vi "writegraph_NEW.vi"(3 "FromPLC":string[][](array[string]), 4 "Numeric":i16, 5 "FromMotes":string[][](array[string])) -> ()   [LabVIEW 2011]
uses:
  Dependencies/global.vi
panel:
  out "Actuation Values":T1(graph)
  out "AC":dbl
  out "Radiator":dbl
  out "FreshAirInlet":dbl
  out "OutdoorTemp":dbl
  out "IndoorTemp":dbl
  out "Humidity":dbl(graph)
  out "Temperature":cluster{"IndoorTemp":dbl, " OutdoorTemp":dbl}(graph)
  out "CO2":dbl(graph)
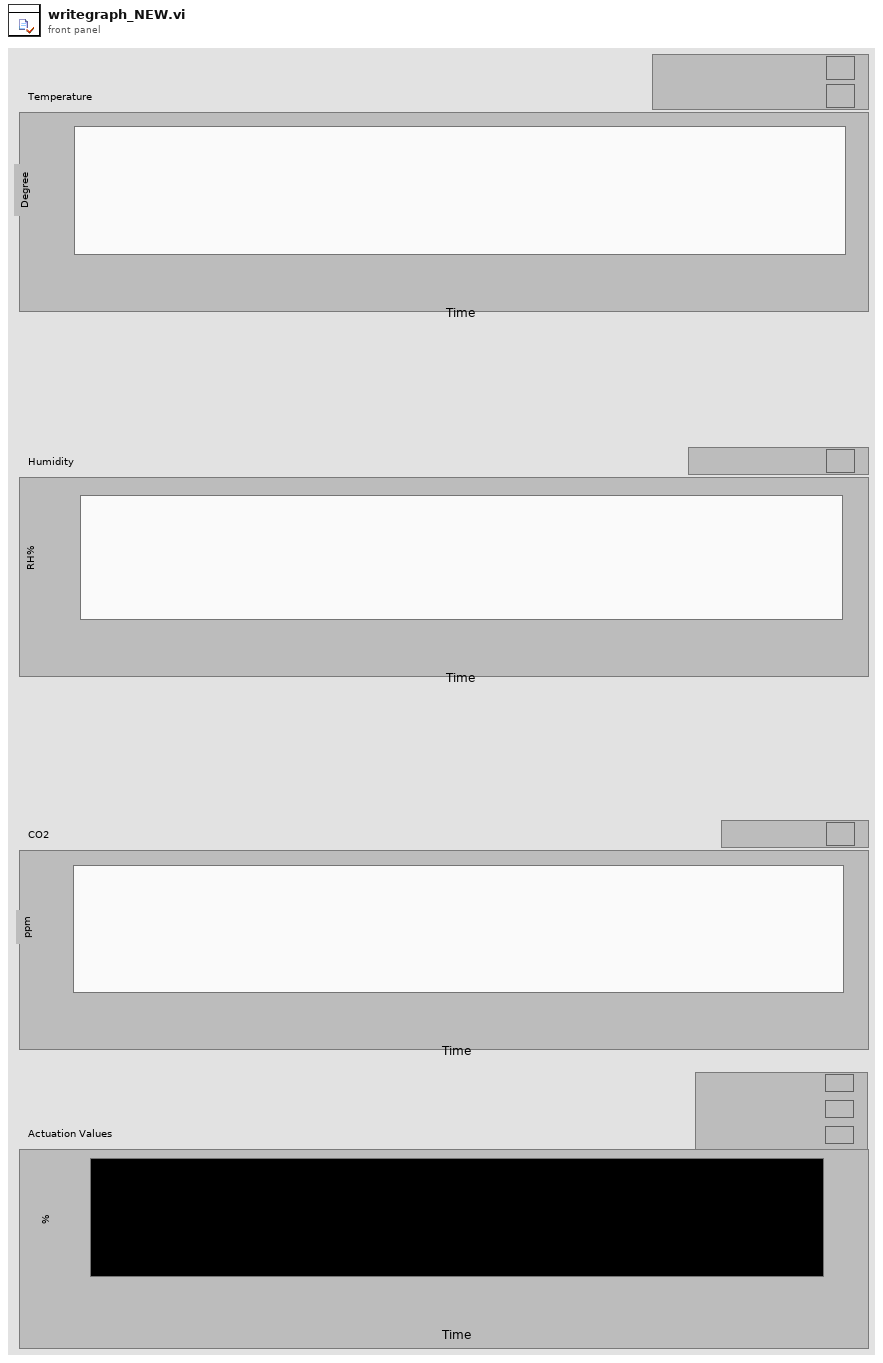
[diagram p1: front panel]
types:
  T1 = cluster{"FreshAirInlet":dbl, "Radiator":dbl, "AC":dbl}
  T2 = typedef "imagedata.ctl" = cluster{"image type":i32, "image depth":i32, "image":u8[], "mask":u8[], "colors":u32[], "Rectangle":cluster{"left":i16, "top":i16, "right":i16, "bottom":i16}}
  T3 = cluster{"FreshAirInlet":dbl, "Radiator":dbl, "AC":dbl}[]
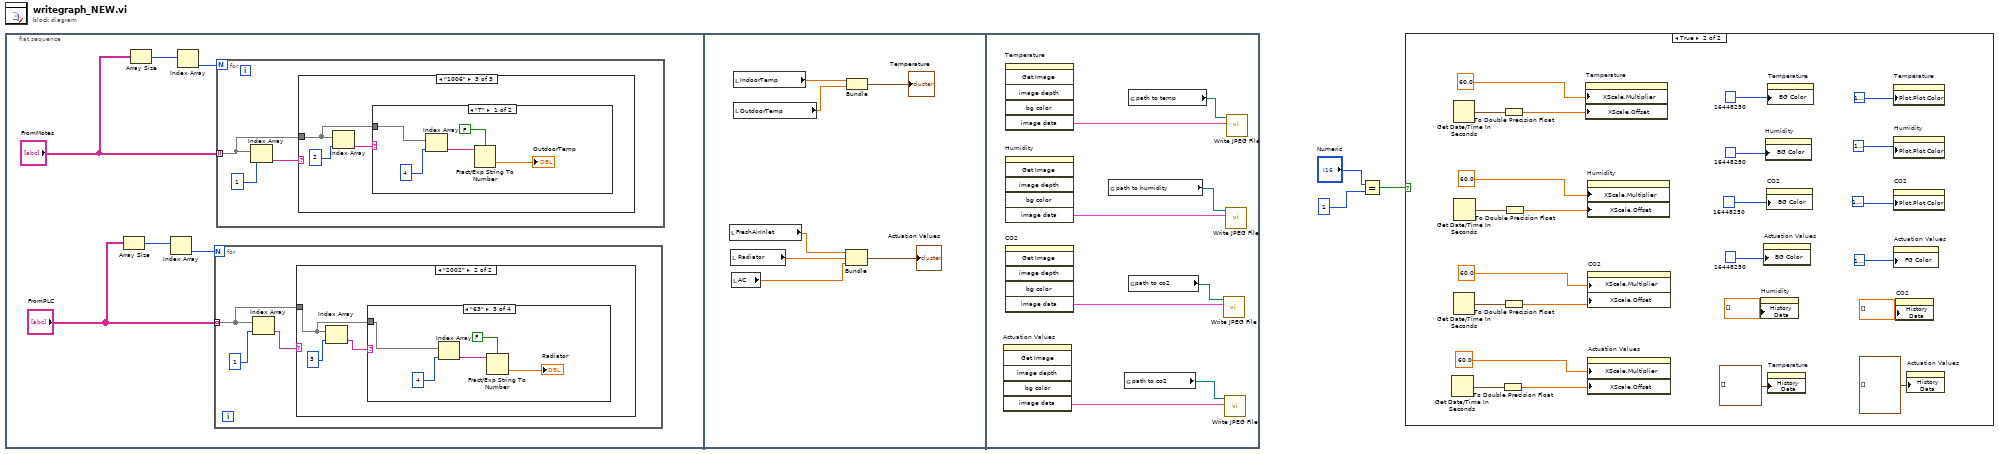
[diagram p0: block diagram]
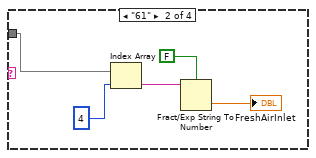
[diagram p4: hidden frame]
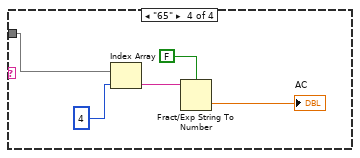
[diagram p5: hidden frame]
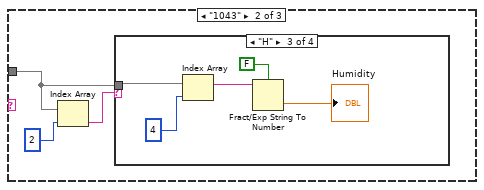
[diagram p7: hidden frame]
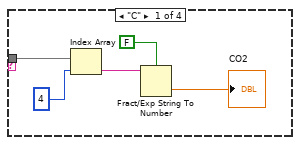
[diagram p8: hidden frame]
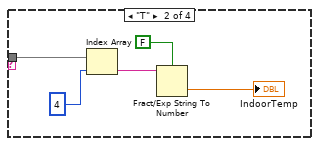
[diagram p9: hidden frame]
diagram:
  n1 = flat-sequence {
    frame #0 {
      n2 = Array Size(array="FromPLC") -> (size(s)=w6:i32[])
      n3 = Array Size(array="FromMotes") -> (size(s)=w9:i32[])
      n4 = Index Array(array=w6) -> (element=w5:i32)  [unwired: 1 in]
      n5 = Index Array(array=w9) -> (element=w8:i32)  [unwired: 1 in]
      n6 = for {
        N: w5 -> [_]
        tunnel: "FromPLC" -> [w10] mode=indexing
        n7 = Index Array(array=w10, index=1) -> (element=w11:string)
        n8 = case shown="\"2002\"" w11 {
          tunnel: w10 -> [_ w13]
          frame "False", Default {
          }
          frame "2002" {
            n9 = Index Array(array=w13, index=3) -> (element=w14:string)
            n10 = case shown="\"63\"" w14 {
              tunnel: w13 -> [_ w17 w22 w27]
              frame Default {
              }
              frame "61" {
                n11 = Index Array(array=w17, index=4 ("index (row)")) -> (element=w19:string)
                n12 = Fract/Exp String To Number(use system decimal point (T)=FALSE, string=w19) -> (number=→"FreshAirInlet":dbl)  [unwired: 2 in, 1 out]
              }
              frame "63" {
                n13 = Index Array(array=w22, index=4 ("index (row)")) -> (element=w24:string)
                n14 = Fract/Exp String To Number(use system decimal point (T)=FALSE, string=w24) -> (number=→"Radiator":dbl)  [unwired: 2 in, 1 out]
              }
              frame "65" {
                n15 = Index Array(array=w27, index=4 ("index (row)")) -> (element=w29:string)
                n16 = Fract/Exp String To Number(use system decimal point (T)=FALSE, string=w29) -> (number=→"AC":dbl)  [unwired: 2 in, 1 out]
              }
            }
          }
        }
      }
      n17 = for {
        N: w8 -> [_]
        tunnel: "FromMotes" -> [w31] mode=indexing
        n18 = Index Array(array=w31, index=1) -> (element=w32:string)
        n19 = case shown="\"1006\"" w32 {
          tunnel: w31 -> [_ w36 w54]
          frame "0", Default {
          }
          frame "1043" {
            n20 = Index Array(array=w36, index=2) -> (element=w34:string)
            n21 = case shown="\"H\"" w34 {
              tunnel: w36 -> [w39 w46 w49 _]
              frame "C" {
                n22 = Index Array(array=w39, index=4 ("index (row)")) -> (element=w40:string)
                n23 = Fract/Exp String To Number(use system decimal point (T)=FALSE, string=w40) -> (number=→"CO2":dbl)  [unwired: 2 in, 1 out]
              }
              frame "T" {
                n24 = Index Array(array=w46, index=4 ("index (row)")) -> (element=w44:string)
                n25 = Fract/Exp String To Number(use system decimal point (T)=FALSE, string=w44) -> (number=→"IndoorTemp":dbl)  [unwired: 2 in, 1 out]
              }
              frame "H" {
                n26 = Index Array(array=w49, index=4 ("index (row)")) -> (element=w50:string)
                n27 = Fract/Exp String To Number(use system decimal point (T)=FALSE, string=w50) -> (number=→"Humidity":dbl)  [unwired: 2 in, 1 out]
              }
              frame Default {
              }
            }
          }
          frame "1006" {
            n28 = Index Array(array=w54, index=2) -> (element=w52:string)
            n29 = case shown="\"T\"" w52 {
              tunnel: w54 -> [w59 _]
              frame "T" {
                n30 = Index Array(array=w59, index=4 ("index (row)")) -> (element=w57:string)
                n31 = Fract/Exp String To Number(use system decimal point (T)=FALSE, string=w57) -> (number=→"OutdoorTemp":dbl)  [unwired: 2 in, 1 out]
              }
              frame Default {
              }
            }
          }
        }
      }
    }
    frame #1 {
      n32 = local read "FreshAirInlet"() -> (w63:dbl)
      n33 = local read "Radiator"() -> (w62:dbl)
      n34 = local read "AC"() -> (w61:dbl)
      n35 = local read "IndoorTemp"() -> (w64:dbl)
      n36 = local read "OutdoorTemp"() -> (w65:dbl)
      n37 = Bundle("FreshAirInlet"=w63, "Radiator"=w62, "AC"=w61) -> (→"Actuation Values":T1)  [unwired: 1 in]
      n38 = Bundle("IndoorTemp"=w64, "OutdoorTemp"=w65) -> (→"Temperature":cluster{"IndoorTemp":dbl, " OutdoorTemp":dbl})  [unwired: 1 in]
    }
    frame #2 {
      n39 = invoke on="Actuation Values" class="WFChart (strict)" method="Get Image"() -> ("image data"=w68:T2)  [unwired: 6 in, 5 out]
      n40 = invoke on="Temperature" class="WFChart (strict)" method="Get Image"() -> ("image data"=w69:T2)  [unwired: 6 in, 5 out]
      n41 = invoke on="Humidity" class="WFChart (strict)" method="Get Image"() -> ("image data"=w70:T2)  [unwired: 6 in, 5 out]
      n42 = invoke on="CO2" class="WFChart (strict)" method="Get Image"() -> ("image data"=w71:T2)  [unwired: 6 in, 5 out]
      n43 = global read "global.vi" "path to humidity"() -> (w73:path)
      n44 = global read "global.vi" "path to co2"() -> (w67:path)
      n45 = global read "global.vi" "path to co2"() -> (w72:path)
      n46 = global read "global.vi" "path to temp"() -> (w74:path)
      n47 = call <vilib>:"Write JPEG File.vi"("image data"=w71, "path to JPEG file"=w72) -> ()  [unwired: 8 in, 2 out]
      n48 = call <vilib>:"Write JPEG File.vi"("image data"=w68, "path to JPEG file"=w67) -> ()  [unwired: 8 in, 2 out]
      n49 = call <vilib>:"Write JPEG File.vi"("image data"=w70, "path to JPEG file"=w73) -> ()  [unwired: 8 in, 2 out]
      n50 = call <vilib>:"Write JPEG File.vi"("image data"=w69, "path to JPEG file"=w74) -> ()  [unwired: 8 in, 2 out]
    }
  }
  n51 = Equal?(x="Numeric", y=i16 1) -> (x = y?=w3:bool)
  n52 = case shown="True" w3 {
    frame False {
    }
    frame True {
      n53 = Get Date/Time In Seconds() -> (seconds since 1Jan1904=w77:timestamp)
      n54 = Get Date/Time In Seconds() -> (seconds since 1Jan1904=w98:timestamp)
      n55 = Get Date/Time In Seconds() -> (seconds since 1Jan1904=w95:timestamp)
      n56 = Get Date/Time In Seconds() -> (seconds since 1Jan1904=w97:timestamp)
      n57 = To Double Precision Float(number=w77) -> (double precision float=w76:dbl)
      n58 = To Double Precision Float(number=w98) -> (double precision float=w92:dbl)
      n59 = To Double Precision Float(number=w95) -> (double precision float=w90:dbl)
      n60 = To Double Precision Float(number=w97) -> (double precision float=w91:dbl)
      n61 = property on="Temperature" class="WFChart (strict)"("XScale.Multiplier"=60.0 ("X Scale.Offset and Multiplier:Multiplier"), "XScale.Offset"=w92) -> ()  [unwired: 2 in, 2 out]
      n62 = property on="Humidity" class="WFChart (strict)"("XScale.Multiplier"=60.0 ("X Scale.Offset and Multiplier:Multiplier"), "XScale.Offset"=w91) -> ()  [unwired: 2 in, 2 out]
      n63 = property on="CO2" class="WFChart (strict)"("XScale.Multiplier"=60.0 ("X Scale.Offset and Multiplier:Multiplier"), "XScale.Offset"=w90) -> ()  [unwired: 2 in, 2 out]
      n64 = property on="Actuation Values" class="WFChart (strict)"("XScale.Multiplier"=60.0 ("X Scale.Offset and Multiplier:Multiplier"), "XScale.Offset"=w76) -> ()  [unwired: 2 in, 2 out]
      n65 = property on="Humidity" class="WFChart (strict)"("History Data"=dbl[] []) -> ()  [unwired: 2 in, 2 out]
      n66 = property on="Actuation Values" class="WFChart (strict)"("BG Color"=u32 16448250) -> ()  [unwired: 2 in, 2 out]
      n67 = property on="Humidity" class="WFChart (strict)"("BG Color"=u32 16448250) -> ()  [unwired: 2 in, 2 out]
      n68 = property on="CO2" class="WFChart (strict)"("BG Color"=u32 16448250) -> ()  [unwired: 2 in, 2 out]
      n69 = property on="Temperature" class="WFChart (strict)"("BG Color"=u32 16448250) -> ()  [unwired: 2 in, 2 out]
      n70 = property on="Temperature" class="WFChart (strict)"("History Data"=cluster{"IndoorTemp":dbl, " OutdoorTemp":dbl}[] []) -> ()  [unwired: 2 in, 2 out]
      n71 = property on="Temperature" class="WFChart (strict)"("Plot.Plot Color"=u32 16777222) -> ()  [unwired: 2 in, 2 out]
      n72 = property on="Humidity" class="WFChart (strict)"("Plot.Plot Color"=u32 16777222) -> ()  [unwired: 2 in, 2 out]
      n73 = property on="CO2" class="WFChart (strict)"("Plot.Plot Color"=u32 16777222) -> ()  [unwired: 2 in, 2 out]
      n74 = property on="Actuation Values" class="WFChart (strict)"("FG Color"=u32 16777222) -> ()  [unwired: 2 in, 2 out]
      n75 = property on="CO2" class="WFChart (strict)"("History Data"=dbl[] []) -> ()  [unwired: 2 in, 2 out]
      n76 = property on="Actuation Values" class="WFChart (strict)"("History Data"=T3 []) -> ()  [unwired: 2 in, 2 out]
    }
  }
